vi "Generate noise.vi"(4 "lo cutoff":dbl, 6 "hi cutoff":dbl, 7 "position noise? (or velocity)":bool, 8 "start amplitude":dbl, 9 "end amplitude":dbl, 10 "sampling freq":dbl, 11 "samples":dbl) -> (3 "noise":dbl[](array[numeric]))   [LabVIEW 2013]
uses:
  <vilib>/Analysis/3filter.llb/Filter Passband Type.ctl
  <vilib>/Analysis/2dsp.llb/Integral Method.ctl
  <vilib>/Analysis/1siggen.llb/Ramp Pattern by Samples.vi
  <vilib>/Analysis/3filter.llb/Butterworth Filter (DBL).vi
  <vilib>/Analysis/NI_AALBase.lvlib
  <vilib>/Analysis/NI_AALPro.lvlib
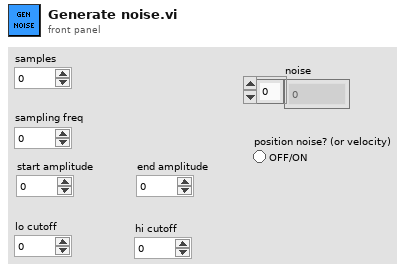
[diagram p1: front panel]
types:
  T1 = typedef "NI_AALBase.lvlib/Filter Passband Type.ctl" = enum32{"Lowpass", "Highpass", "Bandpass", "Bandstop"}
  T2 = typedef "NI_AALPro.lvlib/Integral Method.ctl" = i32
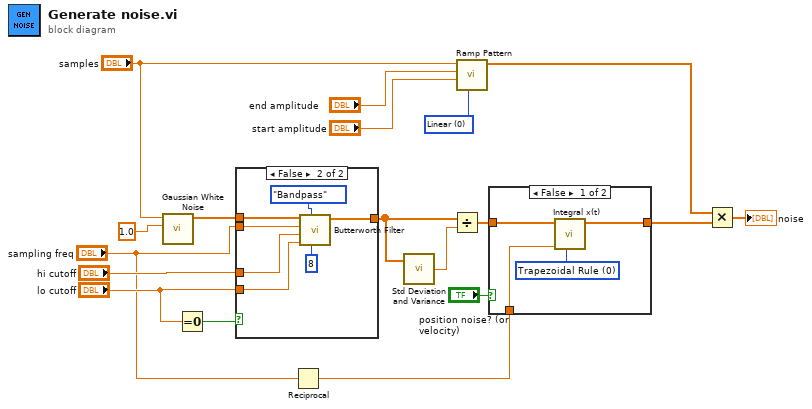
[diagram p0: block diagram]
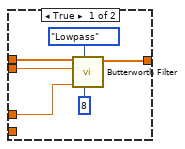
[diagram p3: hidden frame]
diagram:
  w8 = u16 0 items=["Linear", "Logarithmic"] ("type")
  n1 = call <vilib>:"Gaussian White Noise.vi"("standard deviation"=1.0, "samples"="samples") -> ("Gaussian noise pattern"=w17:dbl[])  [unwired: 8 in, 1 out]
  n2 = Equal To 0?(x="lo cutoff") -> (x = 0?=w15:bool)
  n3 = case shown="False" w15 {
    tunnel: "lo cutoff" -> [_ w26]
    tunnel: "hi cutoff" -> [w21 w27]
    tunnel: "sampling freq" -> [w23 w30]
    tunnel: w17 -> [w22 w29]
    tunnel: [w19 w25] -> w13
    frame True {
      n4 = call-poly <vilib>:"Butterworth Filter.vi"("order"=8, "filter type"=Filter_Passband_Type."Lowpass", "low cutoff freq: fl"=w21, "sampling freq: fs"=w23, "X"=w22) -> ("Filtered X"=w19:dbl[])  [unwired: 3 in, 1 out]
    }
    frame False {
      n5 = call-poly <vilib>:"Butterworth Filter.vi"("order"=8, "filter type"=Filter_Passband_Type."Bandpass", "low cutoff freq: fl"=w26, "high cutoff freq: fh"=w27, "sampling freq: fs"=w30, "X"=w29) -> ("Filtered X"=w25:dbl[])  [unwired: 2 in, 1 out]
    }
  }
  n6 = Reciprocal(x="sampling freq") -> (1/x=w2:dbl)
  n7 = call <vilib>:"Std Deviation and Variance.vi"("X"=w13) -> ("standard deviation"=w12:dbl)  [unwired: 1 in, 2 out]
  n8 = Divide(x=w13, y=w12) -> (x/y=w5:dbl[])
  n9 = call-poly <vilib>:"Ramp Pattern.vi"("type"=w8, "start"="start amplitude", "end"="end amplitude", "samples"="samples") -> ("Ramp Pattern"=w7:dbl[])  [unwired: 6 in, 1 out]
  n10 = case shown="False" "position noise? (or velocity)" {
    tunnel: w5 -> [w35 w36]
    tunnel: [w34 w36] -> w4
    tunnel: w2 -> [w33 _]
    frame False {
      w32 = T2 0 items=["Trapezoidal Rule", "Simpson's Rule", "Simpson's 3/8 Rule", "Bode Rule"] ("integration method")
      n11 = call <vilib>:"Integral x(t).vi"("integration method"=w32, "dt"=w33, "X"=w35) -> ("Integral X"=w34:dbl[])  [unwired: 7 in, 1 out]
    }
    frame True {
    }
  }
  n12 = Multiply(x=w7, y=w4) -> (x*y=→"noise":dbl[])
